vi "GetNumericReference.vi"(8 "error in":errorcluster, 11 "Numeric in":refnum<class "Numeric.lvclass">) -> (0 "error out":errorcluster, 1 "Numeric reference":refnum<vi>, 3 "Numeric out":refnum<class "Numeric.lvclass">)   [LabVIEW 2014, in "Raspberry Pi Compatible Compiler for LabVIEW.lvlib" / "Numeric.lvclass"]
uses:
  Numeric.lvclass
  Generic/Generic.lvclass
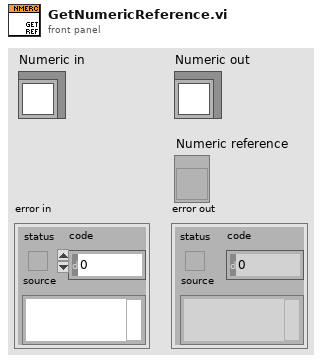
[diagram p1: front panel]
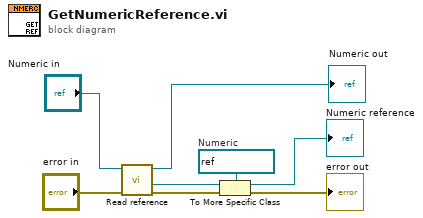
[diagram p0: block diagram]
diagram:
  w8 = refnum<vi> refnum  # Numeric
  n1 = call "Read reference.vi"("error in"="error in", "GObject in"="Numeric in") -> ("error out"=w3:errorcluster, "reference"=w2:refnum<vi>, "GObject out"=→"Numeric out":refnum<class "Numeric.lvclass">)  [unwired: 5 in]
  n2 = To More Specific Class(target class=w8, reference=w2, error in=w3) -> (specific class reference=→"Numeric reference":refnum<vi>, error out=→"error out":errorcluster)
